vi "checkExcel.vi"(0 "reference in":refnum<class "excelFile.lvclass">, 5 "error in (no error)":errorcluster) -> (14 "reference out":refnum<class "excelFile.lvclass">, 19 "error out":errorcluster)   [LabVIEW 2016, in "excelFile.lvclass"]
uses:
  excelFile.lvclass
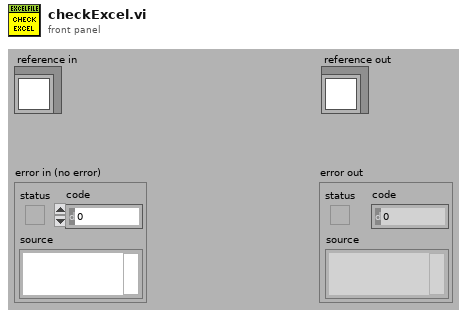
[diagram p1: front panel]
types:
  T1 = typedef "excelFile.lvclass/ObjectAttributesRef.ctl" = refnum<data-value>
  T2 = typedef "excelFile.lvclass/ObjectAttributes.ctl" = cluster{"MyAttribute":dbl, "path":string, "Refnum Excel":cluster{"Excel._Application":refnum<k7>, "Workbooks":refnum<k7>, "Open":refnum<k7>}, "data":string[][][], "save":bool, "fileType":T3, "rowsColor":u32[], "python_ref":refnum<class "python.lvclass">, "items_rows":i32[], "excel_range":i32[][], "TSR":cluster{"number":string, "TSR_path":path, "service_path":path, "email_to":string}, "excel_already_opened?":bool, "file_already_opened?":bool, "excel_protected_opened?":bool}
  T3 = typedef "excelFile.lvclass/fileType.ctl" = enum16{"devices", "items", "partsTracking", "TSR"}
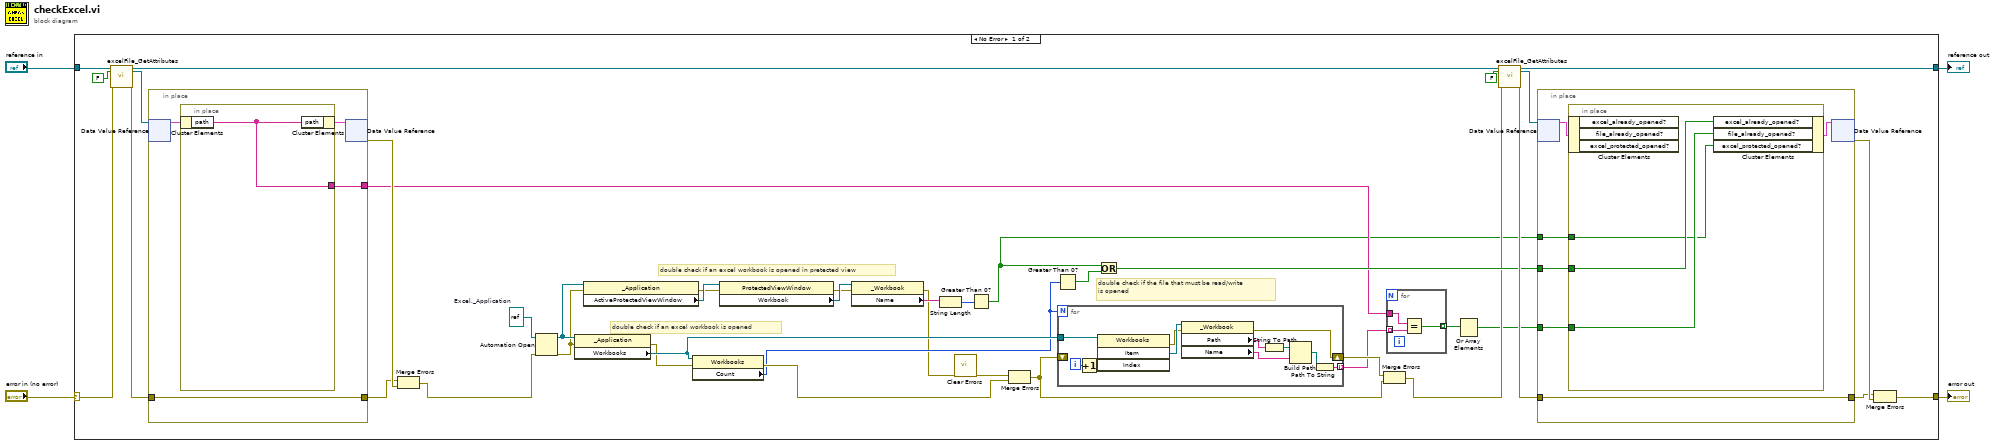
[diagram p0: block diagram]
diagram:
  n1 = case shown="No Error" "error in (no error)" {
    selector: "error in (no error)" -> [w13 w75]
    tunnel: [w39 w75] -> w3
    tunnel: [w41 w74] -> w1
    tunnel: "reference in" -> [w15 w74]
    frame No Error {
      w38 = refnum<k7> refnum  # Excel._Application
      # "double check if the file that must be read/write\nis opened"
      # "double check if an excel workbook is opened"
      # "double check if an excel workbook is opened in pretected view"
      n2 = call "excelFile_GetAttributes.vi"("reference in"=w15, "return data? (T)"=FALSE, "error in (no error)"=w13) -> ("reference out"=w14:refnum<class "excelFile.lvclass">, "attributes ref"=w16:T1, "error out"=w17:errorcluster)  [unwired: 13 in, 1 out]
      n3 = in-place {
        in-place-border: w17 -> [w50]
        in-place-border: [w50] -> w19
        in-place-border: [w49] -> w10
        n4 = in-place-dvr #1(w16) -> (w51:T2)  [unwired: 1 out]
        n5 = in-place {
          in-place-border: [w53] -> w49
          n6 = in-place-cluster #2(w51) -> ("path"=w53:string)
          n7 = in-place-cluster #2("path"=w53) -> (w52:T2)
        }
        n8 = in-place-dvr #1(w52) -> (w20:errorcluster)  [unwired: 1 out]
      }
      n9 = Merge Errors(w19, w20) -> (w12:errorcluster)
      n10 = Automation Open(error in (no error)=w12, Automation Refnum=w38) -> (Automation Refnum=w37:refnum<k7>, error out=w34:errorcluster)  [unwired: 2 in]
      n11 = property class="_Application"(reference=w37, error in=w34) -> (error out=w28:errorcluster, "Workbooks"=w33:refnum<k7>)  [unwired: 1 out]
      n12 = property class="_Application"(reference=w37, error in=w34) -> (error out=w32:errorcluster, "ActiveProtectedViewWindow"=w36:refnum<k7>)  [unwired: 1 out]
      n13 = property class="Workbooks"(reference=w33, error in=w28) -> (error out=w27:errorcluster, "Count"=w26:i32)  [unwired: 1 out]
      n14 = property class="ProtectedViewWindow"(reference=w36, error in=w32) -> (error out=w31:errorcluster, "Workbook"=w35:refnum<k7>)  [unwired: 1 out]
      n15 = property class="_Workbook"(reference=w35, error in=w31) -> (error out=w7:errorcluster, "Name"=w24:string)  [unwired: 1 out]
      n16 = String Length(string=w24) -> (length=w25:i32)
      n17 = call <vilib>:"Clear Errors.vi"("error in (no error)"=w7) -> ("error out"=w6:errorcluster)  [unwired: 5 in, 1 out]
      n18 = Greater Than 0?(x=w25) -> (x > 0?=w5:bool)
      n19 = Merge Errors(w6, w27) -> (w22:errorcluster)
      n20 = Greater Than 0?(x=w26) -> (x > 0?=w30:bool)
      n21 = for {
        N: w26 -> [_]
        tunnel: w33 -> [w64]
        tunnel: [w54] -> w11 mode=indexing
        shift-right: [w59] -> w23
        shift-left: w22 -> [_]
        i -> [w62]
        n22 = Increment(x=w62) -> (x+1=w61:i32)
        n23 = invoke class="Workbooks" method="Item"(reference=w64, "Index"=w61) -> (error out=w60:errorcluster, "Item"=w63:refnum<k7>)  [unwired: 2 in, 2 out]
        n24 = property class="_Workbook"(reference=w63, error in=w60) -> (error out=w59:errorcluster, "Path"=w58:string, "Name"=w57:string)  [unwired: 1 out]
        n25 = String To Path(string=w58) -> (path=w56:path)
        n26 = Build Path(base path=w56, name or relative path=w57) -> (appended path=w55:path)
        n27 = Path To String(path=w55) -> (string=w54:string)
      }
      n28 = Or(x=w5, y=w30) -> (x .or. y?=w29:bool)
      n29 = Merge Errors(w23, w22) -> (w21:errorcluster)
      n30 = for {
        tunnel: w11 -> [w48] mode=indexing
        tunnel: w10 -> [w47]
        tunnel: [w46] -> w9 mode=indexing
        n31 = Equal?(x=w47, y=w48) -> (x = y?=w46:bool)
      }
      n32 = Or Array Elements(Boolean array=w9) -> (logical OR=w8:bool)
      n33 = call "excelFile_GetAttributes.vi"("reference in"=w14, "return data? (T)"=FALSE, "error in (no error)"=w21) -> ("reference out"=w41:refnum<class "excelFile.lvclass">, "attributes ref"=w40:T1, "error out"=w42:errorcluster)  [unwired: 13 in, 1 out]
      n34 = in-place {
        in-place-border: w42 -> [w68]
        in-place-border: [w68] -> w44
        in-place-border: w29 -> [w67]
        in-place-border: w8 -> [w66]
        in-place-border: w5 -> [w65]
        n35 = in-place-dvr #3(w40) -> (w69:T2)  [unwired: 1 out]
        n36 = in-place {
          in-place-border: w67 -> [w73]
          in-place-border: w66 -> [w72]
          in-place-border: w65 -> [w71]
          n37 = in-place-cluster #4(w69) -> ()  [unwired: 3 out]
          n38 = in-place-cluster #4("excel_already_opened?"=w73, "file_already_opened?"=w72, "excel_protected_opened?"=w71) -> (w70:T2)
        }
        n39 = in-place-dvr #3(w70) -> (w45:errorcluster)  [unwired: 1 out]
      }
      n40 = Merge Errors(w44, w45) -> (w39:errorcluster)
    }
    frame Error {
    }
  }
  "error out" <- w3
  "reference out" <- w1
